vi "MQTT_Simple_Connect_and_Subscribe.vi"() -> ()   [LabVIEW 2025, in "DAQIO MQTT.lvlib"]
doc: "A basic client example that connects to a server, subscribes to a variety of topics and receives responses for the topics. \n\n© 2015 - daq.io, LLC - Peter Adelhardt"
uses:
  DAQIO MQTT.lvlib
  Controls/Connection_Return_Codes.ctl
  Controls/DUP_Flag.ctl
  Controls/Retain_Flag.ctl
  Controls/Connect Flags.ctl
  Controls/User Info.ctl
panel:
  out "appended array":cluster{"Topic":string, "Message":string}[](array[cluster])
  in  "Stop Reading":bool
  in  "Subscription Info Array":T1(array[cluster])=[{"Topic"="testtopic/LVMQTT", "QoS"=enum."At most once"}]
  out "Granted QoS Levels":T2(array[ring])
  out "Connection Status":T3=enum."Connection refused: Server unavailable"
  in  "Client ID":string="LVSubscribeClient"
  out "error out":errorcluster
  in  "error in (no error)":errorcluster
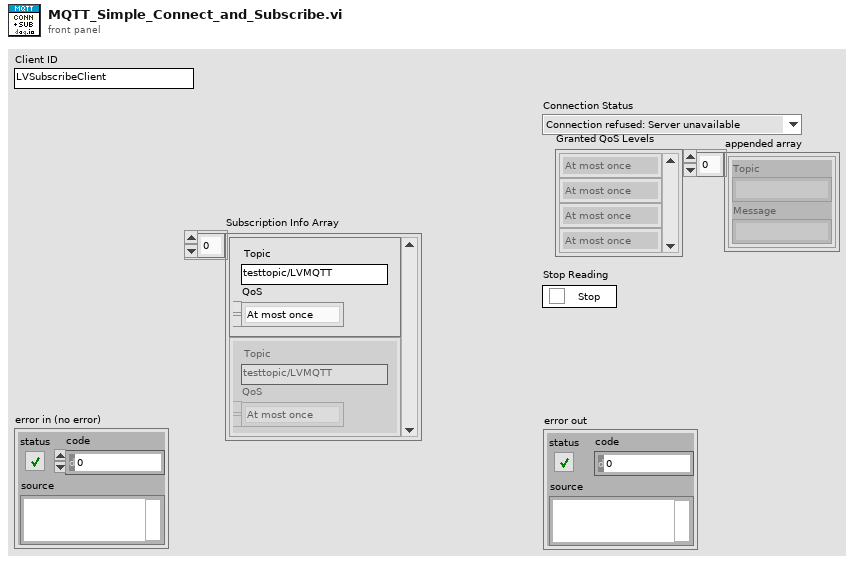
[diagram p1: front panel]
types:
  T1 = cluster{"Topic":string, "QoS":enum8{"At most once", "At least once", "Exactly once", "Reserved"}}[]
  T2 = enum8{"At most once", "At least once", "Exactly once", "Reserved"}[]
  T3 = typedef "DAQIO MQTT.lvlib/Connection_Return_Codes.ctl" = enum16{"Connection accepted", "Connection refused: unacceptable protocol version", "Connection refused: identifier rejected", "Connection refused: Server unavailable", "Connection refused: bad user name or password", "Connection refused: not authorized"}
  T4 = typedef "DAQIO MQTT.lvlib/User Info.ctl" = cluster{"Username":string, "Password":string}
  T5 = typedef "DAQIO MQTT.lvlib/Connect Flags.ctl" = cluster{"user name":bool, "password":bool, "will retain":bool, "will flag":bool, "clean session":bool, "reserved":bool, "will QoS":enum8{"At most once", "At least once", "Exactly once", "Reserved"}}
  T6 = typedef "DAQIO MQTT.lvlib/DUP_Flag.ctl" = bool
  T7 = typedef "DAQIO MQTT.lvlib/Retain_Flag.ctl" = bool
  T8 = cluster{"QoS":enum8{"At most once", "At least once", "Exactly once", "Reserved"}, "DUP":T6, "Retain":T7, "Keep Alive (sec)":u16}
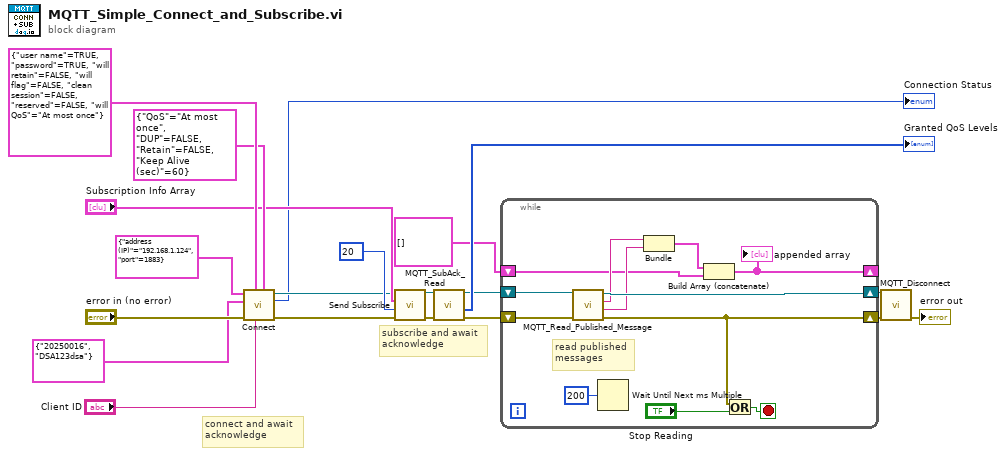
[diagram p0: block diagram]
diagram:
  # "connect and await\nacknowledge"
  # "subscribe and await\nacknowledge"
  n1 = call "Connect.vi"("Connect Meta"=T8 {"QoS"=enum."At most once", "DUP"=FALSE, "Retain"=FALSE, "Keep Alive (sec)"=60}, "Client ID"="Client ID", "Connect Flags"=T5 {"user name"=TRUE, "password"=TRUE, "will retain"=FALSE, "will flag"=FALSE, "clean session"=FALSE, "reserved"=FALSE, "will QoS"=enum."At most once"}, "error in (no error)"="error in (no error)", "User Info"=T4 {"Username"="20250016", "Password"="DSA123dsa"}, "MQTT Broker"=cluster{"address (IP)":string, "port":u16} {"address (IP)"="192.168.1.124", "port"=1883}) -> ("error out"=w3:errorcluster, "Connection Status"=→"Connection Status":T3, "connection ID out"=w5:refnum<k5>)  [unwired: 3 in]
  n2 = call "Send Subscribe.vi"("error in (no error)"=w3, "Message ID"=u16 20, "Subscription Info Array"="Subscription Info Array", "connection ID"=w5) -> ("error out"=w13:errorcluster, "connection ID out"=w14:refnum<k5>)  [unwired: 6 in]
  n3 = call "MQTT_SubAck_Read.vi"("error in (no error)"=w13, "connection ID"=w14) -> ("error out"=w11:errorcluster, "Granted QoS Levels"=→"Granted QoS Levels":T2, "connection ID out"=w10:refnum<k5>)  [unwired: 7 in]
  n4 = while {
    shift-right: [w21] -> _
    shift-left: cluster{"Topic":string, "Message":string}[] [] -> [w23]
    shift-right: [w24] -> w8
    shift-left: w11 -> [w32]
    shift-right: [w30] -> w9
    shift-left: w10 -> [w31]
    stop <- w26 stop-if-true
    # "read published\nmessages"
    n5 = call "MQTT_Read_Published_Message.vi"("error in (no error)"=w32, "connection ID"=w31) -> ("error out"=w24:errorcluster, "Message"=w28:string, "Topic"=w29:string, "connection ID out"=w30:refnum<k5>)  [unwired: 6 in]
    n6 = Wait Until Next ms Multiple(millisecond multiple=u32 200) -> ()  [unwired: 1 out]
    n7 = Bundle("Topic"=w29, "Message"=w28) -> (w22:cluster{"Topic":string, "Message":string})  [unwired: 1 in]
    n8 = Build Array (concatenate)(w22, w23) -> (w21:cluster{"Topic":string, "Message":string}[])
    "appended array" <- w21
    n9 = Or(x=w24, y="Stop Reading") -> (x .or. y?=w26:bool)
  }
  n10 = call "MQTT_Disconnect.vi"("error in (no error)"=w8, "connection ID"=w9) -> ("error out"=→"error out":errorcluster)  [unwired: 9 in]
